vi "Gen_OFDM_Symbol.vi"(4 "EN_CP":dbl, 5 "Nu":dbl, 6 "error in (no error)":errorcluster caption="错误输入（无错误）", 7 "Nsym_slot":dbl, 8 "fredata":cdb[][](array[numeric]), 9 "appended path":path) -> (0 "error IO":errorcluster, 2 "input":cdb[](array[numeric]), 3 "txdata":cdb[](array[numeric]))   [LabVIEW 2015]
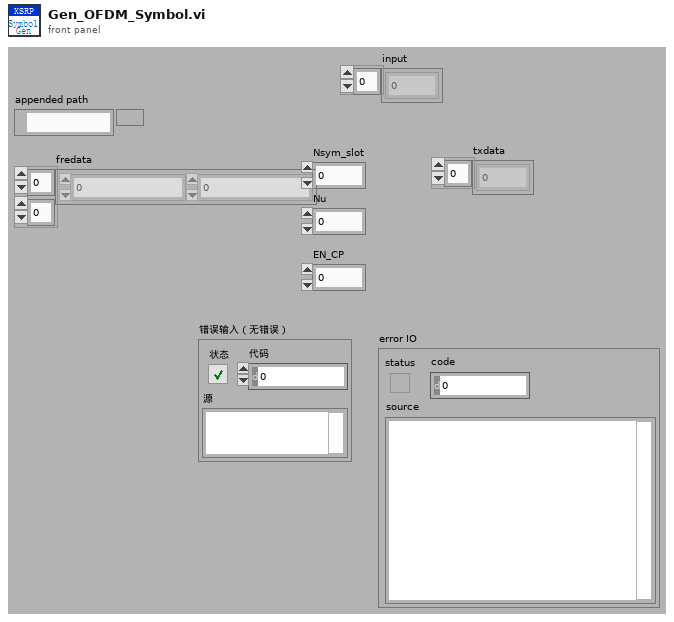
[diagram p1: front panel]
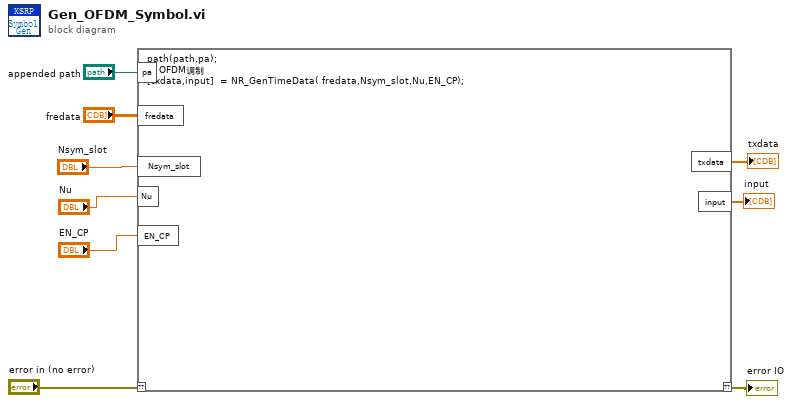
[diagram p0: block diagram]
diagram:
  n1 = script code="path(path,pa);\n% OFDM调制\n[txdata,input]  = NR_GenTimeData( fredata,Nsym_slot,Nu,EN_CP);"("??"="error in (no error)", "pa"="appended path", "fredata"="fredata", "Nsym_slot"="Nsym_slot", "Nu"="Nu", "EN_CP"="EN_CP") -> ("??"=→"error IO":errorcluster, "txdata"=→"txdata":cdb[], "input"=→"input":cdb[])
